vi "WriteToDb.vi"(0 "reference in":refnum<class "Sig_AO.lvclass">, 11 "error in (no error)":errorcluster) -> (4 "reference out":refnum<class "Sig_AO.lvclass">, 15 "error out":errorcluster)   [LabVIEW 2019, in "Sig_AO.lvclass"]
uses:
  Sig_AO.lvclass
  D:/GIT H4000/H4000/src/Proccess_class/Proccess.lvclass
  Proccess_class/Proccess.lvclass/Proccess.ctl
  Sig_AO.lvclass/Sig_AO.ctl
  Logger_class/SignalData.ctl
  TypeDef/engineering units.ctl
  Logger_class/Logger.lvclass/Logger.ctl
  Logger_class/Logger.lvclass
  Proccess_class/Proccess.lvclass
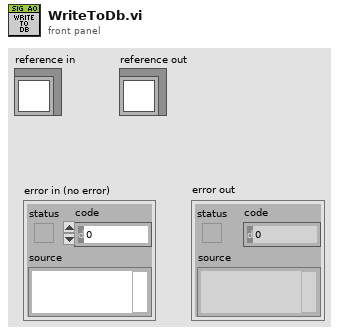
[diagram p1: front panel]
types:
  T1 = typedef "Logger.lvclass/SignalData.ctl" = cluster{"Value":dbl, "SignalTag":string, "ObjTag":string, "engineering units":T2, "Desc":string, "Time Stamp":timestamp}
  T2 = typedef "engineering units.ctl" = enum16{"mV", "V", "mA", "A", "C", "pC", "s", "Pa", "N", "g", "m/s^2", "m/s", "m", "mm/s", "mm", "micron/s", "micron", "in/s^2", "in/s", "in", "mil/s", "mil", "rad/s^2", "rad/s", "rad", "deg/s^2", "deg/s", "deg", "RPM", "cycle/s^2", "Hz", "cycle", "strain", "%"}
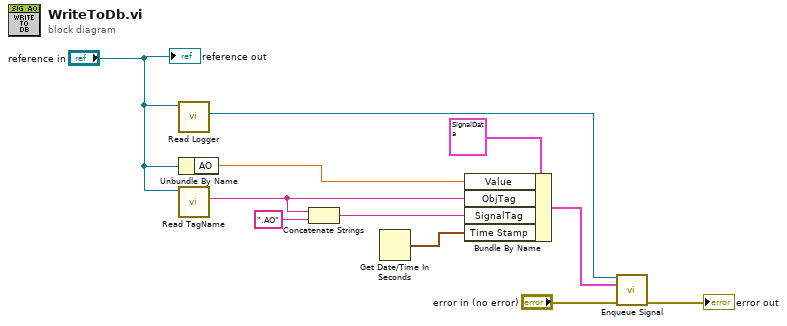
[diagram p0: block diagram]
diagram:
  n1 = call "Read Logger.vi"("Proccess in"="reference in") -> ("Logger"=w2:refnum<class "Logger.lvclass">)  [unwired: 10 in]
  n2 = Unbundle By Name("reference in") -> ("AO"=w6:dbl)
  n3 = call "Read TagName.vi"("Proccess in"="reference in") -> ("TagName"=w3:string)  [unwired: 10 in]
  n4 = Concatenate Strings(w3, ".AO" ("string")) -> (w9:string)
  n5 = Get Date/Time In Seconds() -> (seconds since 1Jan1904=w8:timestamp)
  n6 = Bundle By Name(cluster=T1 {"Value"=0.0, "SignalTag"="", "ObjTag"="", "engineering units"=enum."A", "Desc"="", "Time Stamp"=timestamp(0 s since 1904-01-01)} ("element"), "Value"=w6, "ObjTag"=w3, "SignalTag"=w9, "Time Stamp"=w8) -> (w4:T1)
  n7 = call "Enqueue Signal.vi"("reference in"=w2, "element"=w4, "error in (no error)"="error in (no error)") -> ("error out"=→"error out":errorcluster)  [unwired: 11 in, 1 out]
  "reference out" <- "reference in"
